vi "Write_file_sub_VI.vi"(11 "Output String":string) -> (1 "File Contents":string, 3 "Current VI's path":path)   [LabVIEW 2017]
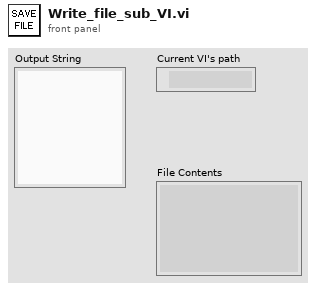
[diagram p1: front panel]
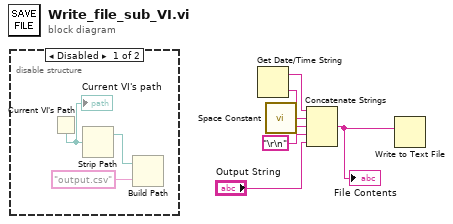
[diagram p0: block diagram]
diagram:
  n1 = disable-structure shown="Disabled" {
    frame Disabled {
      n2 = Current VI's Path() -> (path=w7:path)
      "Current VI's path" <- w7
      n3 = Strip Path(path=w7) -> (stripped path=w8:path)  [unwired: 1 out]
      n4 = Build Path(base path=w8, name or relative path="output.csv") -> ()  [unwired: 1 out]
    }
    frame Enabled {
    }
  }
  n5 = Get Date/Time String() -> (date string=w1:string, time string=w2:string)  [unwired: 3 in]
  n6 = call <vilib>:"Space Constant.vi"() -> ("String"=w4:string)
  n7 = Concatenate Strings(w1, w4, w2, "\r\n", "Output String") -> (w6:string)
  "File Contents" <- w6
  n8 = Write to Text File(text=w6) -> ()  [unwired: 3 in, 3 out]
